vi "GetPWM.vi"(8 "error in (no error)":errorcluster, 9 "Off":bool, 10 "Led num":u8, 11 "PCA in":refnum<class "PCA.lvclass">) -> (0 "error out":errorcluster, 2 "PWM Led N":u8, 3 "PCA out":refnum<class "PCA.lvclass">)   [LabVIEW 2022 SP3, in "PCA9685.lvlib" / "PCA.lvclass"]
uses:
  PCA.lvclass
  PCA.lvclass/PCA.ctl
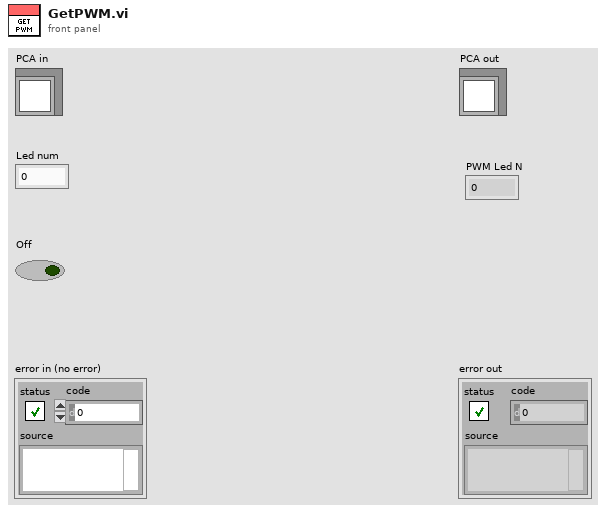
[diagram p1: front panel]
types:
  T1 = typedef "PCA9685.lvlib/PCA.lvclass/Led.ctl" = cluster{"Led_onL":i8, "Led_onH":i8, "Led_offL":i8, "Led_offH":i8}
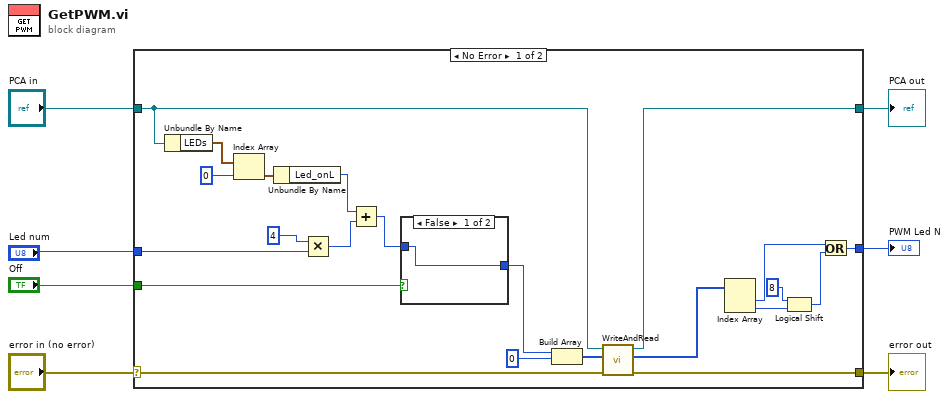
[diagram p0: block diagram]
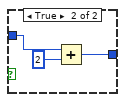
[diagram p2: hidden frame]
diagram:
  n1 = case shown="No Error" "error in (no error)" {
    selector: "error in (no error)" -> [w29 w35]
    tunnel: [w28 w35] -> w6
    tunnel: [w14 w34] -> w4
    tunnel: "PCA in" -> [w15 w34]
    tunnel: "Led num" -> [w22 _]
    tunnel: "Off" -> [w20 _]
    tunnel: [w8 _] -> w1
    frame No Error {
      n2 = Unbundle By Name(w15) -> ("LEDs"=w27:T1[])
      n3 = Index Array(array=w27, index=0) -> (element=w25:T1)
      n4 = Unbundle By Name(w25) -> ("Led_onL"=w24:i8)
      n5 = Multiply(x=i8 4 ("y"), y=w22) -> (x*y=w21:u8)
      n6 = Add(x=w24, y=w21) -> (x+y=w18:u8)
      n7 = case shown="False" w20 {
        tunnel: w18 -> [w30 w33]
        tunnel: [w30 w31] -> w16
        frame False {
        }
        frame True {
          n8 = Add(x=w33, y=u8 2) -> (x+y=w31:u8)
        }
      }
      n9 = Build Array(w16, u8 0 ("element")) -> (w17:u8[])
      n10 = call "WriteAndRead.vi"("error in (no error)"=w29, "Data"=w17, "PCA in"=w15) -> ("error out"=w28:errorcluster, "Data 2"=w13:u8[], "PCA out"=w14:refnum<class "PCA.lvclass">)  [unwired: 6 in]
      n11 = Index Array(array=w13) -> (element #1=w12:u8, element #2=w11:u8)  [unwired: 2 in]
      n12 = Logical Shift(y=i16 8, x=w11) -> (x << y=w9:u8)
      n13 = Or(x=w12, y=w9) -> (x .or. y?=w8:u8)
    }
    frame Error {
    }
  }
  "error out" <- w6
  "PCA out" <- w4
  "PWM Led N" <- w1
